vi "JsonFile Save.vi"(6 "Pretty Print(T)":bool=TRUE, 8 "error in (no error)":errorcluster, 10 "JSON String":string, 11 "Path":path) -> (0 "error out":errorcluster)   [LabVIEW 2019, in "lv-apt-json-file.lvlib"]
uses:
  lv-apt-json-file.lvlib
  <vilib>/Utility/error.llb/Clear Errors.vi
  Json/Remove Comments.vi
  <userlib>/NEVSTOP-Programming-Palette/Configuration/Ini/TextToLines.vi
  <userlib>/_OpenG.lib/array/array.llb/Filter 1D Array__ogtk.vi
  <userlib>/_OpenG.lib/array/array.llb/Filter 1D Array (U8)__ogtk.vi
  <userlib>/NEVSTOP-Programming-Palette/Configuration/Ini/LinesToText.vi
  <vilib>/addons/_JKI.lib/Serialization/JSON/Library/Unflatten From JSON String.vi
  <vilib>/Utility/error.llb/Error Cluster From Error Code.vi
  <userlib>/FTools/JSON Pretty Printer/JSON Pretty Printer.lvlib
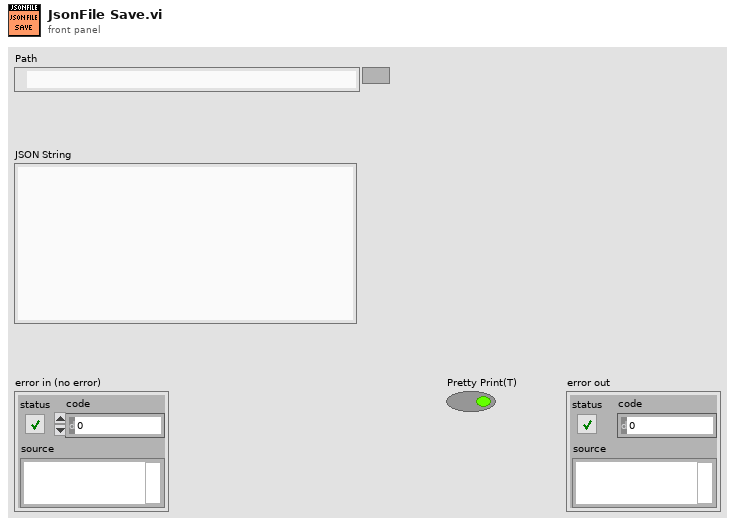
[diagram p1: front panel]
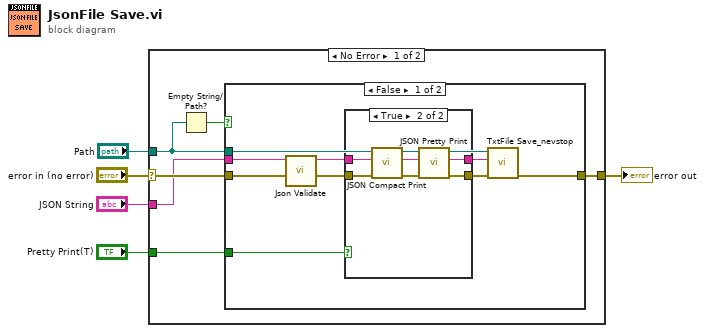
[diagram p0: block diagram]
diagram:
  n1 = case shown="No Error" "error in (no error)" {
    selector: "error in (no error)" -> [w9 w30]
    tunnel: [w11 w30] -> w5
    tunnel: "Path" -> [w8 _]
    tunnel: "JSON String" -> [w7 _]
    tunnel: "Pretty Print(T)" -> [w6 _]
    frame No Error {
      n2 = Empty String/Path?(string/path=w8) -> (empty?=w10:bool)
      n3 = case shown="False" w10 {
        tunnel: w9 -> [w17 w29]
        tunnel: [w20 w29] -> w11
        tunnel: w7 -> [w18 _]
        tunnel: w8 -> [w19 _]
        tunnel: w6 -> [w12 _]
        frame False {
          n4 = call "Json Validate.vi"("error in (no error)"=w17, "String"=w18) -> ("error out"=w14:errorcluster, "Json without comments"=w16:string)  [unwired: 6 in, 2 out]
          n5 = case shown="True" w12 {
            tunnel: w16 -> [w22 w26]
            tunnel: [w22 w25] -> w15
            tunnel: w14 -> [w21 w24]
            tunnel: [w21 w23] -> w13
            frame False {
            }
            frame True {
              n6 = call <userlib>:"JSON Compact Print.vi"("error in"=w24, "JSON Pretty String"=w26) -> ("error out"=w27:errorcluster, "JSON Compact String"=w28:string)  [unwired: 8 in]
              n7 = call <userlib>:"JSON Pretty Print.vi"("error in"=w27, "JSON String"=w28) -> ("error out"=w23:errorcluster, "JSON Pretty Print Format"=w25:string)  [unwired: 8 in]
            }
          }
          n8 = call <userlib>:"TxtFile Save_nevstop.vi"("error in (no error)"=w13, "text"=w15, "Path"=w19) -> ("error out"=w20:errorcluster)  [unwired: 8 in]
        }
        frame True {
        }
      }
    }
    frame Error {
    }
  }
  "error out" <- w5
